vi "Test Process Multiple Init.vi"(8 "error in (no error)":errorcluster, 11 "Process Test In":refnum<class "Process Test.lvclass">) -> (0 "error out":errorcluster, 3 "Process Test Out":refnum<class "Process Test.lvclass">)   [LabVIEW 2020, in "Process Test.lvclass"]
uses:
  Process Test.lvclass
  C:/Program Files (x86)/National Instruments/LabVIEW 2020/vi.lib/Asteme/LUnit/Test Case.lvclass
  Mock Error Handler/Mock Error Handler.lvclass
  C:/Users/anton/Documents/GitHub/Triarc-Framework/source/Framework/Process/Process.lvclass
  C:/Users/anton/Documents/GitHub/Triarc-Framework/source/Framework/Error Handler Interface/Error Handler Interface.lvclass
  Framework/Process/Process.lvclass/Process.ctl
  <vilib>/Asteme/LUnit/Test Case.lvclass/Test Case.ctl
  <vilib>/Asteme/LUnit/LUnit Assertion Result.lvclass/LUnit Assertion Result.ctl
  Framework/Process/Public/Get Lifecycle State.vi
  Framework/Process/Protected/Messaging/Enqueue Message.vi
  <vilib>/Utility/error.llb/Clear Errors.vi
  <vilib>/Asteme/LUnit/Palette/Fail.vi
  <vilib>/Asteme/LUnit/Palette/Pass.vi
  <vilib>/Asteme/LUnit/Set Assertion Type.vi
  <vilib>/Asteme/LUnit/Variant to string.vi
  Framework/Process/Private/SubVIs/Wait for finish.vi
  Framework/Process/Private/SubVIs/Set Lifecycle State.vi
  <vilib>/Asteme/LUnit/Add test result.vi
  <vilib>/Asteme/LUnit/LUnit Write Passed.vi
  <vilib>/Asteme/LUnit/LUnit Get Test Case.vi
  <vilib>/Asteme/LUnit/LUnit Write Message.vi
  <vilib>/Asteme/LUnit/LUnit Write Description.vi
  <vilib>/Asteme/LUnit/LUnit Write Assertion Type.vi
  <vilib>/Asteme/LUnit/Read Test Case Name.vi
  <vilib>/Utility/error.llb/Error Cluster From Error Code.vi
  <vilib>/Asteme/LUnit/Assertion Result/LUnit Get Test Name.vi
  <vilib>/Utility/Data Type/Get Type Information.vi
  <vilib>/Utility/LVClass/Get LV Class Name.vi
  Framework/Process/Process.lvclass
  <vilib>/Asteme/LUnit/LUnit Assertion Result.lvclass
  <vilib>/Asteme/LUnit/Test Case.lvclass
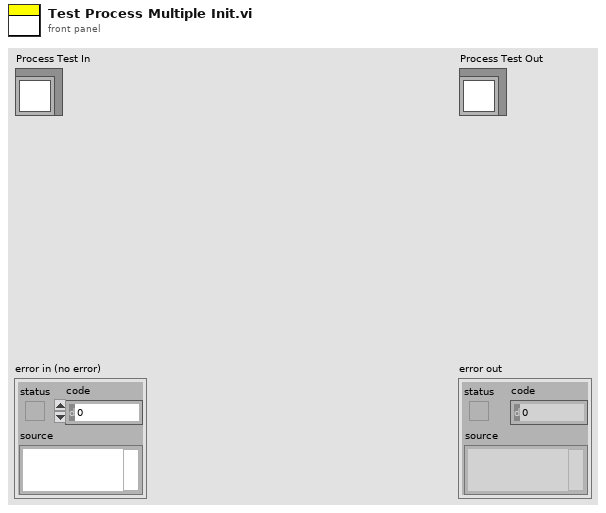
[diagram p1: front panel]
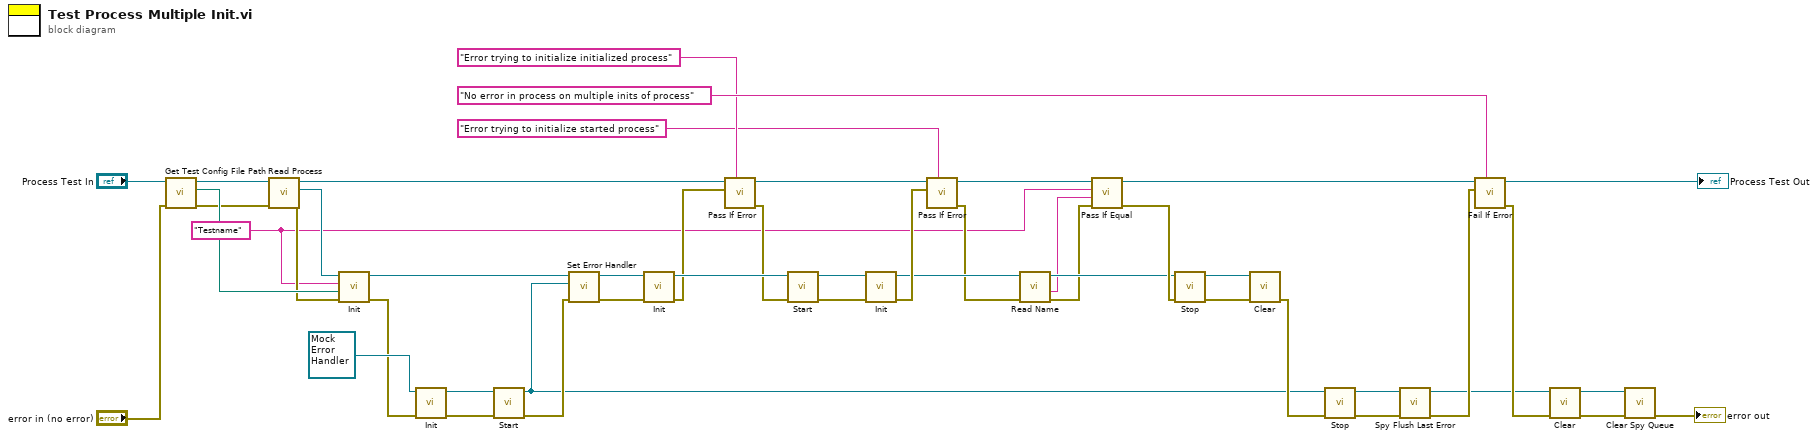
[diagram p0: block diagram]
diagram:
  w1 = "Testname" ("Name")
  n1 = call-dynamic "Get Test Config File Path.vi"("error in (no error)"="error in (no error)", "Base Class Test in"="Process Test In") -> ("error out"=w40:errorcluster, "Test config path"=w43:path, "Base Class Test out"=w45:refnum<class "Process Test.lvclass">)  [unwired: 7 in]
  n2 = call "Read Process.vi"("error in (no error)"=w40, "Process Test in"=w45) -> ("error out"=w41:errorcluster, "Process.lvclass"=w42:refnum<class "Process.lvclass">, "Process Test out"=w16:refnum<class "Process Test.lvclass">)  [unwired: 7 in]
  n3 = call-dynamic "Init.vi"("error in (no error)"=w41, "Config File Path"=w43, "Name"=w1, "Process In"=w42) -> ("error out"=w31:errorcluster, "Process Out"=w46:refnum<class "Process.lvclass">)  [unwired: 6 in]
  n4 = call-dynamic "Init.vi"("error in (no error)"=w31, "Mock Error Handler In"=refnum<class "Mock Error Handler.lvclass"> refnum ("Mock Error Handler.lvclass")) -> ("error out"=w35:errorcluster, "Mock Error Handler Out"=w34:refnum<class "Mock Error Handler.lvclass">)  [unwired: 8 in]
  n5 = call "Start.vi"("error in (no error)"=w35, "Process In"=w34) -> ("error out"=w30:errorcluster, "Process Out"=w21:refnum<class "Mock Error Handler.lvclass">)  [unwired: 8 in]
  n6 = call "Set Error Handler.vi"("error in (no error)"=w30, "Error Handler"=w21, "Process In"=w46) -> ("error out"=w36:errorcluster, "Process Out"=w37:refnum<class "Process.lvclass">)  [unwired: 7 in]
  n7 = call-dynamic "Init.vi"("error in (no error)"=w36, "Process In"=w37) -> ("error out"=w14:errorcluster, "Process Out"=w48:refnum<class "Process.lvclass">)  [unwired: 8 in]
  n8 = call <vilib>:"Pass If Error.vi"("Description"="Error trying to initialize initialized process", "Assert error"=w14, "Test Case In"=w16) -> ("error out"=w13:errorcluster, "Test Case Out"=w8:refnum<class "Process Test.lvclass">)  [unwired: 7 in]
  n9 = call "Start.vi"("error in (no error)"=w13, "Process In"=w48) -> ("error out"=w15:errorcluster, "Process Out"=w10:refnum<class "Process.lvclass">)  [unwired: 8 in]
  n10 = call-dynamic "Init.vi"("error in (no error)"=w15, "Process In"=w10) -> ("error out"=w11:errorcluster, "Process Out"=w9:refnum<class "Process.lvclass">)  [unwired: 8 in]
  n11 = call <vilib>:"Pass If Error.vi"("Description"="Error trying to initialize started process", "Assert error"=w11, "Test Case In"=w8) -> ("error out"=w4:errorcluster, "Test Case Out"=w7:refnum<class "Process Test.lvclass">)  [unwired: 7 in]
  n12 = call-dynamic "Read Name.vi"("error in (no error)"=w4, "Process In"=w9) -> ("error out"=w3:errorcluster, "Name"=w2:string, "Process Out"=w5:refnum<class "Process.lvclass">)  [unwired: 6 in, 1 out]
  n13 = call <vilib>:"Pass If Equal.vi"("error in (no error)"=w3, "Actual"=w2, "Expected"=w1, "Test Case In"=w7) -> ("error out"=w17:errorcluster, "Test Case Out"=w18:refnum<class "Process Test.lvclass">)  [unwired: 6 in]
  n14 = call "Stop.vi"("error in (no error)"=w17, "Process In"=w5) -> ("error out"=w38:errorcluster, "Process Out"=w39:refnum<class "Process.lvclass">)  [unwired: 7 in, 1 out]
  n15 = call-dynamic "Clear.vi"("error in (no error)"=w38, "Process In"=w39) -> ("error out"=w29:errorcluster)  [unwired: 8 in, 1 out]
  n16 = call "Stop.vi"("error in (no error)"=w29, "Process In"=w21) -> ("error out"=w26:errorcluster, "Process Out"=w22:refnum<class "Mock Error Handler.lvclass">)  [unwired: 7 in, 1 out]
  n17 = call "Spy Flush Last Error.vi"("error in (no error)"=w26, "Mock Error Handler In"=w22) -> ("error out"=w28:errorcluster, "Mock Error Handler Out"=w25:refnum<class "Mock Error Handler.lvclass">)  [unwired: 6 in, 2 out]
  n18 = call <vilib>:"Fail If Error.vi"("Description"="No error in process on multiple inits of process", "Assert error"=w28, "Test Case In"=w18) -> ("error out"=w27:errorcluster, "Test Case Out"=→"Process Test Out":refnum<class "Process Test.lvclass">)  [unwired: 7 in]
  n19 = call-dynamic "Clear.vi"("error in (no error)"=w27, "Process In"=w25) -> ("error out"=w23:errorcluster, "Process Out"=w24:refnum<class "Mock Error Handler.lvclass">)  [unwired: 8 in]
  n20 = call-dynamic "Clear Spy Queue.vi"("error in (no error)"=w23, "Mock Process In"=w24) -> ("error out"=→"error out":errorcluster)  [unwired: 8 in, 1 out]
